vi "PZT Z scan.vi"(8 "error in":errorcluster, 10 "PZT step":i16, 11 "Coarse Approach.lvclass":refnum<class "Coarse Approach.lvclass">) -> (0 "error out":errorcluster, 1 "Z voltage":i16, 2 "x >= y?":bool, 3 "Coarse Approach.lvclass":refnum<class "Coarse Approach.lvclass">)   [LabVIEW 2020, in "Coarse Approach.lvclass"]
uses:
  Coarse Approach.lvclass
  Coarse Approach.lvclass/Coarse Approach.ctl
  PZT/PZT.lvclass
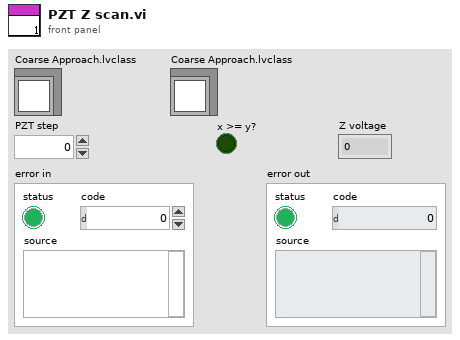
[diagram p1: front panel]
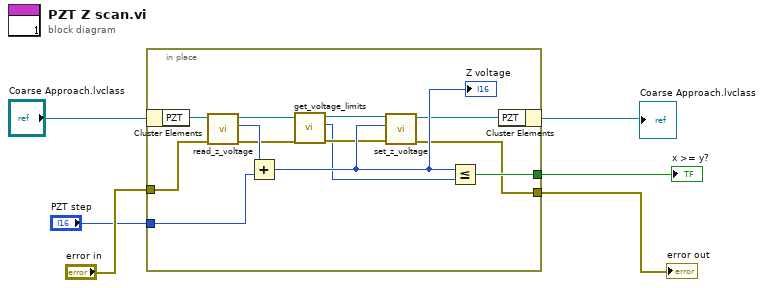
[diagram p0: block diagram]
diagram:
  n1 = in-place {
    in-place-border: "error in" -> [w19]
    in-place-border: [w13] -> w4
    in-place-border: [w17] -> w2
    in-place-border: "PZT step" -> [w15]
    n2 = in-place-cluster #1("Coarse Approach.lvclass") -> ("PZT"=w18:refnum<class "PZT.lvclass">)
    n3 = call "read_z_voltage.vi"("error in"=w19, "PZT in"=w18) -> ("error out"=w10:errorcluster, "Z Voltage out"=w16:i16, "PZT out"=w11:refnum<class "PZT.lvclass">)  [unwired: 7 in]
    n4 = Add(x=w16, y=w15) -> (x+y=w14:i16)
    "Z voltage" <- w14
    n5 = call-dynamic "get_voltage_limits.vi"("error in (no error)"=w10, "PZT in"=w11) -> ("error out"=w8:errorcluster, "maximum voltage (bits)"=w7:i16, "PZT out"=w9:refnum<class "PZT.lvclass">)  [unwired: 6 in, 1 out]
    n6 = call-dynamic "set_z_voltage.vi"("error in (no error)"=w8, "Z voltage (bits)"=w14, "PZT in"=w9) -> ("error out"=w13:errorcluster, "PZT out"=w12:refnum<class "PZT.lvclass">)  [unwired: 7 in]
    n7 = Less Or Equal?(x=w14, y=w7) -> (x <= y?=w17:bool)
    n8 = in-place-cluster #1("PZT"=w12) -> (→"Coarse Approach.lvclass":refnum<class "Coarse Approach.lvclass">)
  }
  "error out" <- w4
  "x >= y?" <- w2
